vi "find VI recursively.vi"(7 "VIs Name":string[](array[string]), 8 "error in (no error)":errorcluster, 10 "Project Item":refnum<vi>[](array[refnum]), 11 "VI Ref In":path[](array[path])) -> (0 "error out":errorcluster, 3 "VI Ref Out":path[](array[path]), 5 "VIs Name Out":string[](array[string]))   [LabVIEW 2023, in "Adjust FP VIs.lvlib"]
doc: "Find VI Recursively."
uses:
  Adjust FP VIs.lvlib
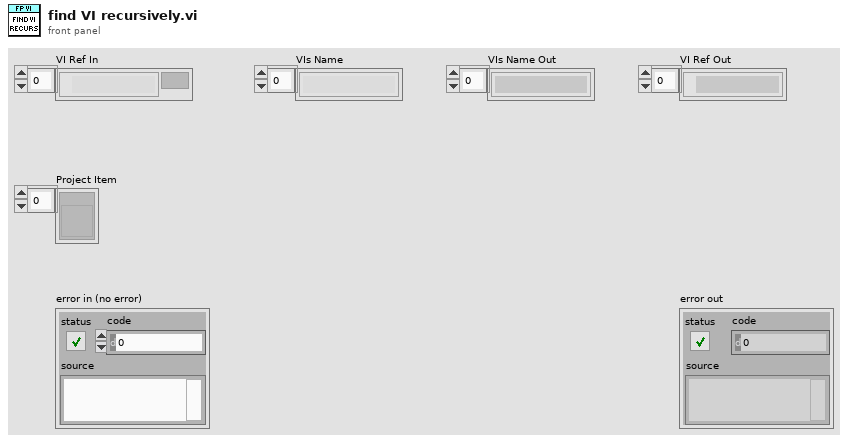
[diagram p1: front panel]
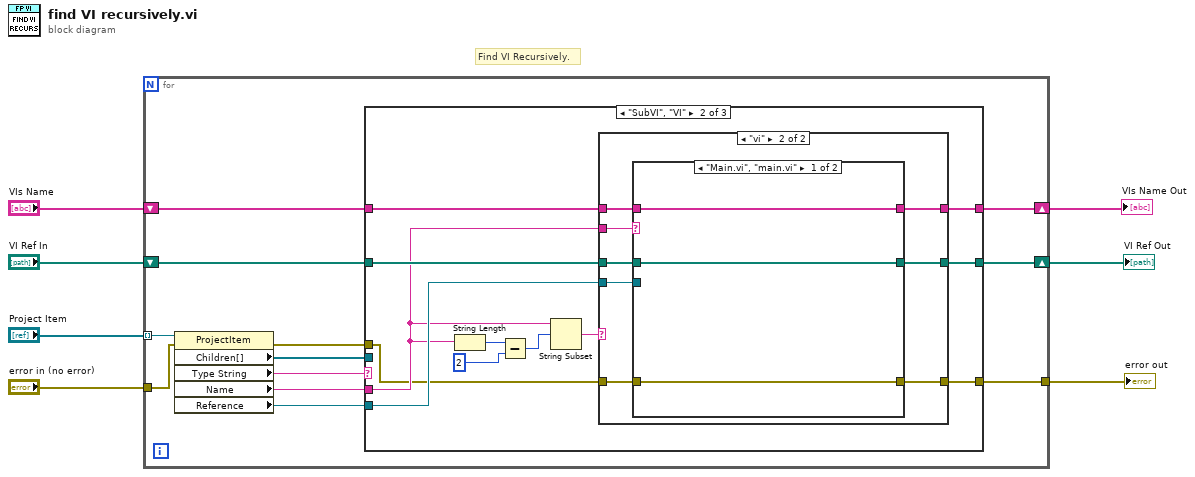
[diagram p0: block diagram]
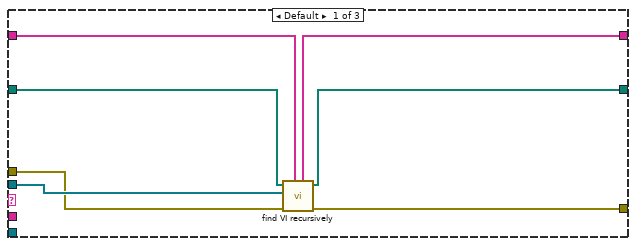
[diagram p2: hidden frame]
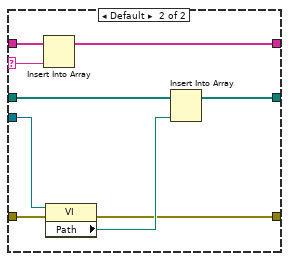
[diagram p4: hidden frame]
diagram:
  # "Find VI Recursively."
  n1 = for {
    tunnel: "Project Item" -> [w19] mode=indexing
    shift-right: [w14] -> w5
    shift-left: "VIs Name" -> [w15]
    shift-right: [w11] -> w3
    shift-left: "VI Ref In" -> [w13]
    tunnel: [w10] -> w2
    tunnel: "error in (no error)" -> [w9]
    n2 = property on="Property Node" class="ProjectItem"(reference=w19, error in=w9) -> (error out=w12:errorcluster, "Children[]"=w17:refnum<vi>[], "Type String"=w18:string, "Name"=w16:string, "Reference"=w8:refnum<vi>)  [unwired: 1 out]
    n3 = case shown="\"SubVI\", \"VI\"" w18 {
      tunnel: w17 -> [w24 _ _]
      tunnel: w16 -> [_ w33 _]
      tunnel: w15 -> [w26 w38 w64]
      tunnel: [w25 w37 w64] -> w14
      tunnel: w13 -> [w23 w36 w63]
      tunnel: w12 -> [w21 w28 w62]
      tunnel: [w22 w35 w63] -> w11
      tunnel: [w20 w27 w62] -> w10
      tunnel: w8 -> [_ w34 _]
      frame Default {
        n4 = call "find VI recursively.vi"("VIs Name"=w26, "error in (no error)"=w21, "Project Item"=w24, "VI Ref In"=w23) -> ("error out"=w20:errorcluster, "VI Ref Out"=w22:path[], "VIs Name Out"=w25:string[])  [unwired: 5 in]
      }
      frame "SubVI", "VI" {
        n5 = String Length(string=w33) -> (length=w32:i32)
        n6 = Subtract(x=w32, y=2) -> (x-y=w30:i32)
        n7 = String Subset(string=w33, offset (0)=w30) -> (substring=w29:string)  [unwired: 1 in]
        n8 = case shown="\"vi\"" w29 {
          tunnel: w38 -> [w41 w49]
          tunnel: [w41 w48] -> w37
          tunnel: w36 -> [w40 w47]
          tunnel: [w40 w46] -> w35
          tunnel: w34 -> [_ w45]
          tunnel: w33 -> [_ w44]
          tunnel: w28 -> [w39 w43]
          tunnel: [w39 w42] -> w27
          frame Default {
          }
          frame "vi" {
            n9 = case shown="\"Main.vi\", \"main.vi\"" w44 {
              selector: w44 -> [_ w57]
              tunnel: w49 -> [w52 w61]
              tunnel: [w52 w60] -> w48
              tunnel: w47 -> [w51 w59]
              tunnel: [w51 w58] -> w46
              tunnel: w45 -> [_ w56]
              tunnel: w43 -> [w50 w54]
              tunnel: [w50 w53] -> w42
              frame "Main.vi", "main.vi" {
              }
              frame Default {
                n10 = Insert Into Array(array=w61, new element=w57) -> (w60:string[])  [unwired: 1 in]
                n11 = property class="VI"(reference=w56, error in=w54) -> (error out=w53:errorcluster, "Path"=w55:path)  [unwired: 1 out]
                n12 = Insert Into Array(array=w59, new element=w55) -> (w58:path[])  [unwired: 1 in]
              }
            }
          }
        }
      }
      frame "Build", "Dependencies" {
      }
    }
  }
  "VIs Name Out" <- w5
  "VI Ref Out" <- w3
  "error out" <- w2
